vi "File Select Multiple Patterns.vi"(5 "Button Label":string, 7 "Prompt":string, 8 "error in":errorcluster, 9 "File Selector Settings":T1(array[cluster])=[{"File Type Selector Label"="ESBR Files", "Array of File Filters"=["BR*.BIN", "BR*.bin"]}, {"File Type Selector Label"="ESBR and ESFI Files", "Array of File Filters"=["BR*.BIN", "BR*.bin", "FI*.BIN", "FI*.bin"]}], 10 "Default Name":string, 11 "Start Path":path=path "") -> (0 "error out":errorcluster, 1 "Cancelled":bool, 2 "Exists":bool, 3 "Selected Path":path)   [LabVIEW 2017]
doc: "This VI will create a browse dialog which allows for multiple selection types with patterns defined by <b>File Selector Settings</b>. This dialog will be to select a single New or Existing File."
panel:
  # "#VIA_Ignore Array Default Values"
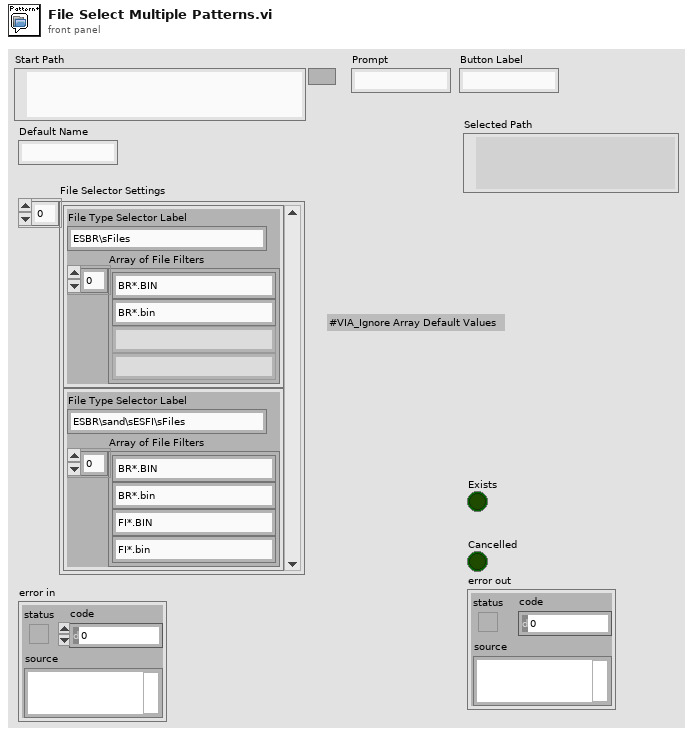
[diagram p1: front panel]
types:
  T1 = cluster{"File Type Selector Label":string, "Array of File Filters":string[]}[]
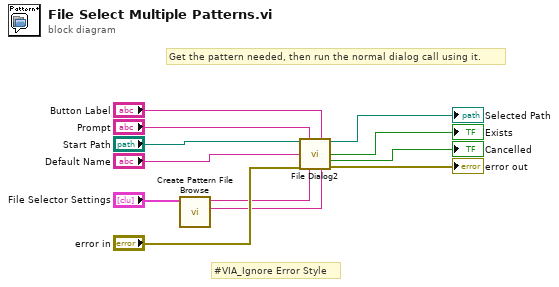
[diagram p0: block diagram]
diagram:
  # "#VIA_Ignore Error Style"
  # "Get the pattern needed, then run the normal dialog call using it."
  n1 = call "Create Pattern File Browse.vi"("File Selector Settings"="File Selector Settings") -> ("Pattern Label"=w2:string, "Pattern"=w3:string)  [unwired: 9 in]
  n2 = call "File Dialog2"("start path"="Start Path", "prompt"="Prompt", "button label"="Button Label", "default name"="Default Name", "error in"="error in", "pattern (all files)"=w3, "pattern label"=w2) -> ("selected path"=→"Selected Path":path, "exists"=→"Exists":bool, "cancelled"=→"Cancelled":bool, "error out"=→"error out":errorcluster)  [unwired: 5 in]
